vi "Config FM Step Increment.vi"(0 "VISA Resource Name":refnum<visa-resource-name>, 5 "Path (0:1)":enum16{"1", "2"}(ring), 7 "Internal Frequency (0: UP)":i16(ring) items=["UP", "DOWN"], 9 "Frequency Step (1.0)":dbl=1.0, 11 "error in (no error)":errorcluster {"code" format="%.0x"}) -> (4 "VISA Resource Name Out":refnum<visa-resource-name>, 15 "error out":errorcluster {"code" format="%.0x"})   [LabVIEW 2014, in "Agilent ESG Series.lvlib"]
doc: "This VI configures FM Step Increment parameters.\n\nNotes:\n(1) This VI is supported for Agilent E4438C only."
uses:
  Agilent ESG Series.lvlib
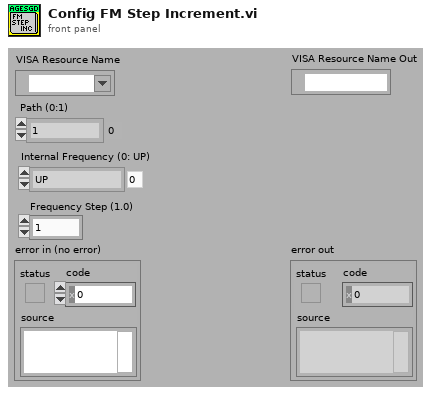
[diagram p1: front panel]
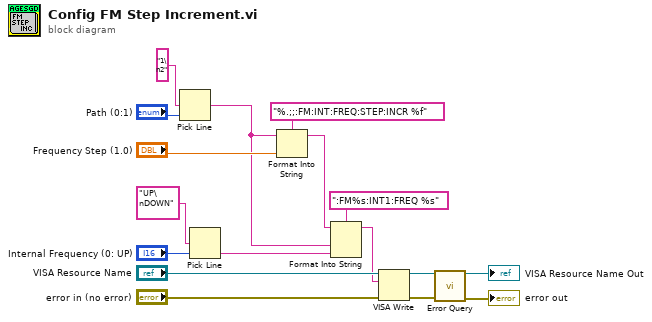
[diagram p0: block diagram]
diagram:
  n1 = Pick Line(multi-line string="1\n2", line index="Path (0:1)") -> (output string=w1:string)  [unwired: 1 in]
  n2 = Pick Line(multi-line string="UP\nDOWN", line index="Internal Frequency (0: UP)") -> (output string=w8:string)  [unwired: 1 in]
  n3 = Format Into String(format string="%.;;:FM:INT:FREQ:STEP:INCR %f", initial string=w1, "Frequency Step (1.0)") -> (resulting string=w2:string)  [unwired: 1 in, 1 out]
  n4 = Format Into String(format string=":FM%s:INT1:FREQ %s", initial string=w2, w1, w8) -> (resulting string=w4:string)  [unwired: 1 in, 1 out]
  n5 = VISA Write(VISA resource name="VISA Resource Name", write buffer=w4, error in (no error)="error in (no error)") -> (VISA resource name out=w13:refnum<visa-resource-name>, error out=w12:errorcluster)  [unwired: 1 out]
  n6 = call "Error Query.vi"("VISA Resource Name"=w13, "error in (no error)"=w12) -> ("VISA Resource Name Out"=→"VISA Resource Name Out":refnum<visa-resource-name>, "error out"=→"error out":errorcluster)  [unwired: 10 in, 2 out]
